vi "GetPartsinPartStudio.vi"(8 "error in":errorcluster, 11 "Device In":T1) -> (0 "error out":errorcluster, 1 "id":string, 2 "documentMicroversion":string, 3 "Device Out":T1)   [LabVIEW 2019]
uses:
  <userlib>/IoT Devices/_subVIs/HTTPComm.ctl
  <userlib>/Onshape/_SubVI/Cluster.ctl
panel:
  out "Comm":T2
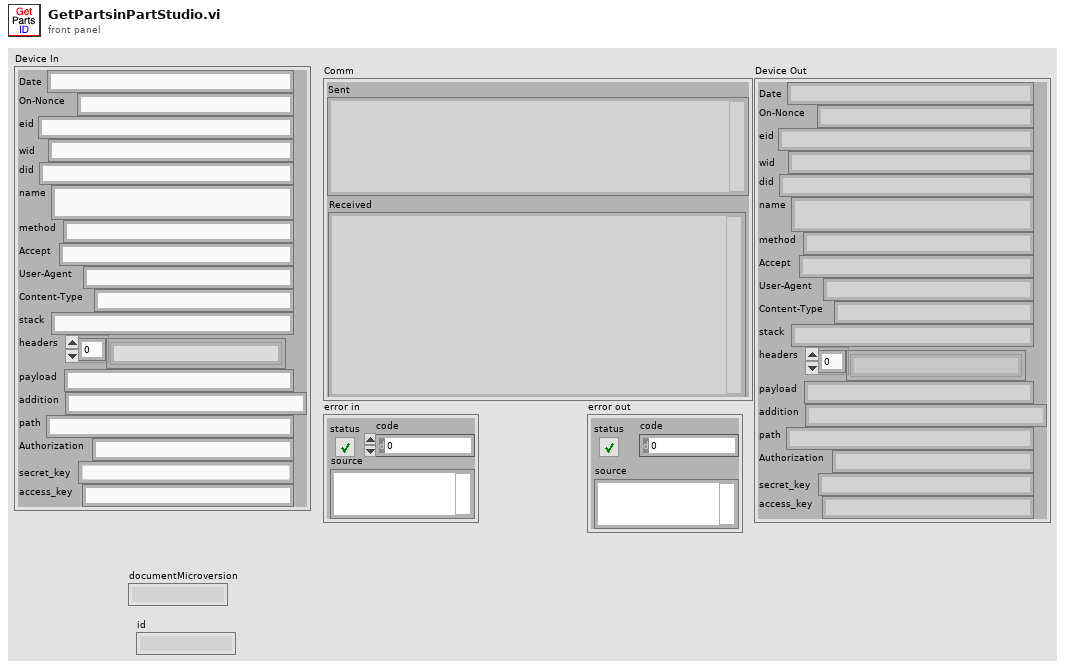
[diagram p1: front panel]
types:
  T1 = typedef "Cluster.ctl" = cluster{"Date":string, "On-Nonce":string, "eid":string, "wid":string, "did":string, "name":string, "method":string, "Accept":string, "User-Agent":string, "Content-Type":string, "stack":string, "headers":string[], "payload":string, "addition":string, "path":string, "Authorization":string, "secret_key":string, "access_key":string}
  T2 = typedef "HTTPComm.ctl" = cluster{"url":string, "sent headers":string, "sent body":string, "headers":string, "body":string, "Sent":string, "Received":string}
  T3 = cluster{"bodies":cluster{"faces":cluster{"id":string, "surface":cluster{"normal":dbl[], "type":string}}[]}[], "documentMicroversion":string}
  T4 = cluster{"faces":cluster{"id":string, "surface":cluster{"normal":dbl[], "type":string}}[]}[]
  T5 = cluster{"faces":cluster{"id":string, "surface":cluster{"normal":dbl[], "type":string}}[]}
  T6 = cluster{"id":string, "surface":cluster{"normal":dbl[], "type":string}}[]
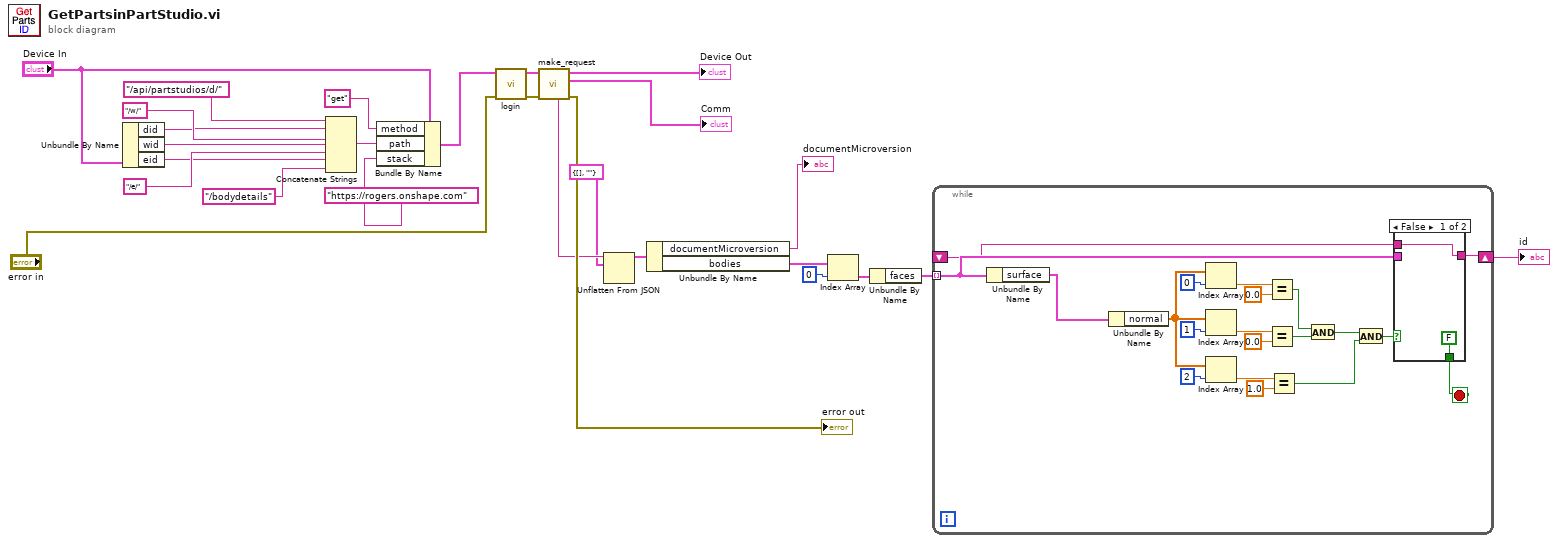
[diagram p0: block diagram]
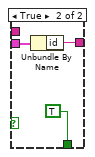
[diagram p2: hidden frame]
diagram:
  n1 = Unbundle By Name("Device In") -> ("did"=w17:string, "wid"=w16:string, "eid"=w15:string)
  n2 = Concatenate Strings("/api/partstudios/d/" ("payload"), w17, "/w/" ("string"), w16, "/e/" ("string"), w15, "/bodydetails" ("string")) -> (w23:string)
  n3 = Bundle By Name(cluster="Device In", "method"="get" ("Method"), "path"=w23, "stack"="https://rogers.onshape.com" ("stacks")) -> (w13:T1)
  n4 = call <userlib>:"login.vi"("error in"="error in", "Device In"=w13) -> ("error out"=w19:errorcluster, "Device Out"=w21:T1)  [unwired: 8 in]
  n5 = call <userlib>:"make_request.vi"("Error in"=w19, "Device In"=w21) -> ("error out"=→"error out":errorcluster, "Comm"=→"Comm":T2, "Device Out"=→"Device Out":T1, "body"=w12:string)  [unwired: 5 in, 1 out]
  n6 = Unflatten From JSON(JSON string=w12, type and defaults=T3 {"bodies"=[], "documentMicroversion"=""}) -> (value=w7:T3)  [unwired: 5 in, 1 out]
  n7 = Unbundle By Name(w7) -> ("documentMicroversion"=→"documentMicroversion":string, "bodies"=w6:T4)
  n8 = Index Array(array=w6, index=0) -> (element=w4:T5)
  n9 = Unbundle By Name(w4) -> ("faces"=w2:T6)
  n10 = while {
    tunnel: w2 -> [w46] mode=indexing
    shift-right: [w45] -> w1
    shift-left: _ -> [w44]
    stop <- w43 stop-if-true
    n11 = Unbundle By Name(w46) -> ("surface"=w47:cluster{"normal":dbl[], "type":string})
    n12 = Unbundle By Name(w47) -> ("normal"=w42:dbl[])
    n13 = Index Array(array=w42, index=0) -> (element=w38:dbl)
    n14 = Index Array(array=w42, index=1) -> (element=w37:dbl)
    n15 = Index Array(array=w42, index=2) -> (element=w35:dbl)
    n16 = Equal?(x=w38, y=0.0) -> (x = y?=w32:bool)
    n17 = Equal?(x=w37, y=0.0) -> (x = y?=w31:bool)
    n18 = Equal?(x=w35, y=1.0) -> (x = y?=w29:bool)
    n19 = And(x=w32, y=w31) -> (x .and. y?=w30:bool)
    n20 = And(x=w30, y=w29) -> (x .and. y?=w28:bool)
    n21 = case shown="False" w28 {
      tunnel: w46 -> [_ w52]
      tunnel: [w49 w51] -> w45
      tunnel: w44 -> [w49 _]
      tunnel: [FALSE TRUE] -> w43
      frame False {
      }
      frame True {
        n22 = Unbundle By Name(w52) -> ("id"=w51:string)
      }
    }
  }
  "id" <- w1
